vi "物料信息录入.vi"(0 "物料名称":string, 1 "功能":enum16{"录入", "清空"}(ring), 5 "物料编码":string, 11 "错误输入（无错误）":errorcluster) -> (15 "错误输出":errorcluster)   [LabVIEW 2018]
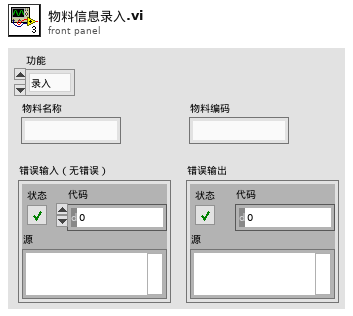
[diagram p1: front panel]
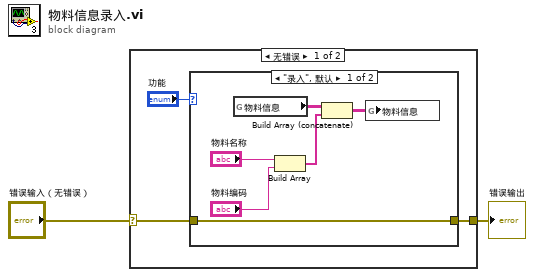
[diagram p0: block diagram]
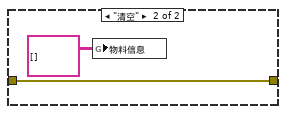
[diagram p2: hidden frame]
diagram:
  n1 = case shown="无错误" "错误输入（无错误）" {
    selector: "错误输入（无错误）" -> [w4 w14]
    tunnel: [w3 w14] -> w1
    frame No Error {
      n2 = case shown="\"录入\", 默认" "功能" {
        tunnel: [w6 w13] -> w3
        tunnel: w4 -> [w6 w13]
        frame "录入", Default {
          n3 = global read "追溯全部变量.vi" "物料信息"() -> (w8:string[][])
          n4 = Build Array("物料名称", "物料编码") -> (w11:string[])
          n5 = Build Array (concatenate)(w8, w11) -> (w7:string[][])
          n6 = global write "追溯全部变量.vi" "物料信息"(w7) -> ()
        }
        frame "清空" {
          n7 = global write "追溯全部变量.vi" "物料信息"(string[][] [] ("物料信息")) -> ()
        }
      }
    }
    frame Error {
    }
  }
  "错误输出" <- w1
